vi "Logout.vi"(8 "error in (no error)":errorcluster, 11 "Person in":refnum<class "Person.lvclass">) -> (0 "error out":errorcluster, 3 "Person out":refnum<class "Person.lvclass">)   [LabVIEW 2014, in "Person.lvclass"]
uses:
  Person.lvclass
  Person.lvclass/Person.ctl
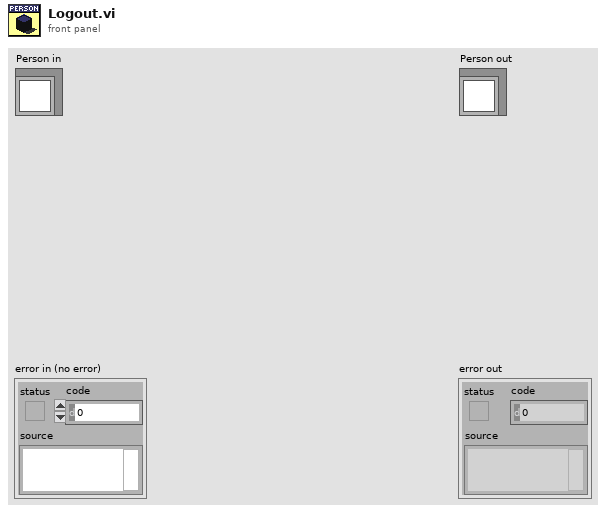
[diagram p1: front panel]
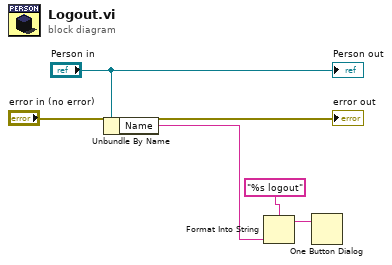
[diagram p0: block diagram]
diagram:
  n1 = Unbundle By Name("Person in") -> ("Name"=w3:string)
  n2 = Format Into String(format string="%s logout", w3) -> (resulting string=w4:string)  [unwired: 2 in, 1 out]
  n3 = One Button Dialog(message=w4) -> ()  [unwired: 1 in, 1 out]
  "error out" <- "error in (no error)"
  "Person out" <- "Person in"
